vi "Untitled 2.vi"() -> ()   [LabVIEW 2019]
panel:
  out "output cluster 2":T1 {"Slide" scale=0.0..10.0}
  out "output cluster":cluster{"Boolean":bool, "Slide":dbl}
  out "Boolean":bool
  out "Numeric":dbl
  in  "stop":bool
  in  "Cluster":T1 {"Slide" scale=0.0..10.0}
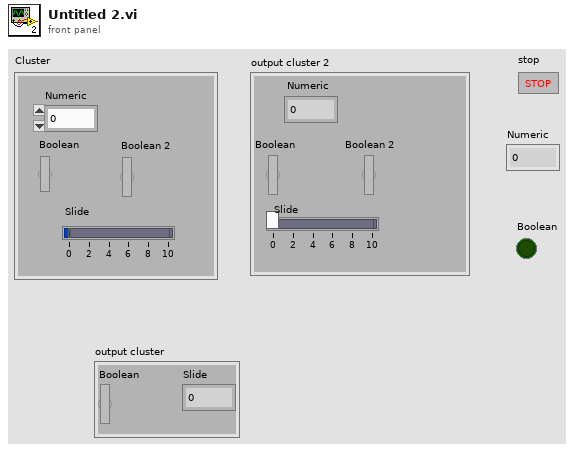
[diagram p1: front panel]
types:
  T1 = cluster{"Numeric":dbl, "Boolean":bool, "Boolean 2":bool, "Slide":dbl}
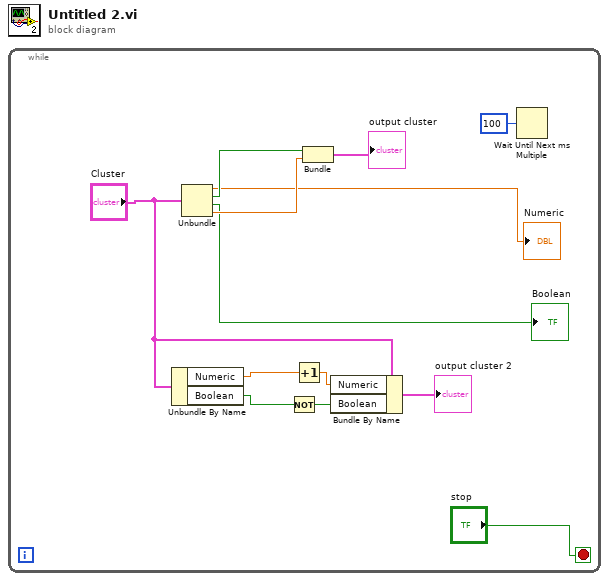
[diagram p0: block diagram]
diagram:
  n1 = while {
    stop <- "stop" stop-if-true
    n2 = Unbundle By Name("Cluster") -> ("Numeric"=w7:dbl, "Boolean"=w6:bool)
    n3 = Unbundle("Cluster") -> ("Numeric"=→"Numeric":dbl, "Boolean"=w13:bool, "Boolean 2"=→"Boolean":bool, "Slide"=w12:dbl)
    n4 = Not(x=w6) -> (.not. x?=w5:bool)
    n5 = Increment(x=w7) -> (x+1=w4:dbl)
    n6 = Bundle("Boolean"=w13, "Slide"=w12) -> (→"output cluster":cluster{"Boolean":bool, "Slide":dbl})  [unwired: 1 in]
    n7 = Bundle By Name(cluster="Cluster", "Numeric"=w4, "Boolean"=w5) -> (→"output cluster 2":T1)
    n8 = Wait Until Next ms Multiple(millisecond multiple=u32 100) -> ()  [unwired: 1 out]
  }
